vi "WPI_DashboardUpdateNames.vi"(11 "Controls on Tab":refnum<vi>[](array[refnum])) -> ()   [LabVIEW 2025]
doc: "Compare and update the captions, displayed names, of the controls on the Basic Tab. The names can be modified directly by editing on the panel, or they can be set in robot code such as is shown in Begin.vi."
uses:
  <vilib>/Rock Robotics/Network Tables/NT Read String Array.vi
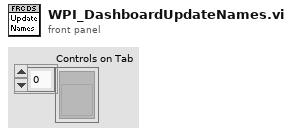
[diagram p1: front panel]
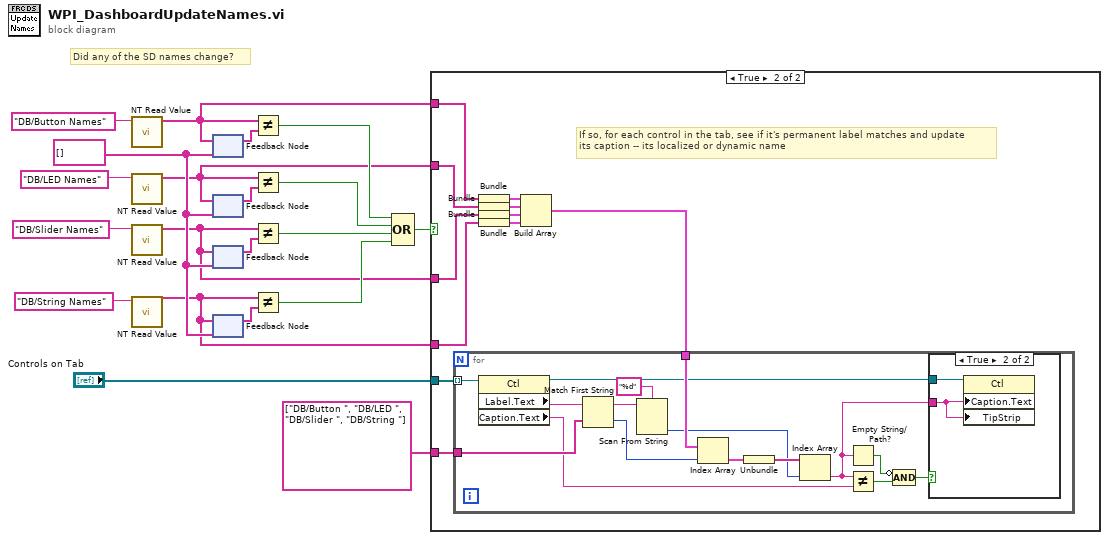
[diagram p0: block diagram]
diagram:
  w13 = string[] []
  # "Did any of the SD names change?"
  n1 = call-poly <vilib>:"NT Read Value.vi"("name"="DB/Button Names" ("Name")) -> ("value"=w7:string[])  [unwired: 8 in, 2 out]
  n2 = call-poly <vilib>:"NT Read Value.vi"("name"="DB/LED Names" ("Name")) -> ("value"=w2:string[])  [unwired: 8 in, 2 out]
  n3 = call-poly <vilib>:"NT Read Value.vi"("name"="DB/Slider Names" ("Name")) -> ("value"=w3:string[])  [unwired: 8 in, 2 out]
  n4 = call-poly <vilib>:"NT Read Value.vi"("name"="DB/String Names" ("Name")) -> ("value"=w6:string[])  [unwired: 8 in, 2 out]
  n5 = feedback #1(w13) -> (w14:string[])
  n6 = feedback-in #1(w7) -> ()
  n7 = feedback-in #2(w2) -> ()
  n8 = feedback #2(w13) -> (w20:string[])
  n9 = feedback #3(w13) -> (w19:string[])
  n10 = feedback-in #3(w3) -> ()
  n11 = feedback #4(w13) -> (w18:string[])
  n12 = feedback-in #4(w6) -> ()
  n13 = Not Equal?(x=w7, y=w14) -> (x != y?=w12:bool)
  n14 = Not Equal?(x=w2, y=w20) -> (x != y?=w11:bool)
  n15 = Not Equal?(x=w3, y=w19) -> (x != y?=w9:bool)
  n16 = Not Equal?(x=w6, y=w18) -> (x != y?=w10:bool)
  n17 = Compound Arithmetic op=OR(w12, w11, w9, w10) -> (w17:bool)
  n18 = case shown="True" w17 {
    tunnel: "Controls on Tab" -> [_ w31]
    tunnel: string[] ["DB/Button ", "DB/LED ", "DB/Slider ", "DB/String "] -> [_ w30]
    tunnel: w7 -> [_ w22]
    tunnel: w2 -> [_ w23]
    tunnel: w6 -> [_ w24]
    tunnel: w3 -> [_ w25]
    frame False {
    }
    frame True {
      # "If so, for each control in the tab, see if it's permanent label matches and update\nits caption -- its localized or dynamic name"
      n19 = Bundle("value"=w22) -> (w29:cluster{"value":string[]})  [unwired: 1 in]
      n20 = Bundle("value"=w23) -> (w28:cluster{"value":string[]})  [unwired: 1 in]
      n21 = Bundle("value"=w25) -> (w27:cluster{"value":string[]})  [unwired: 1 in]
      n22 = Bundle("value"=w24) -> (w26:cluster{"value":string[]})  [unwired: 1 in]
      n23 = Build Array(w29, w28, w27, w26) -> (w21:cluster{"value":string[]}[])
      n24 = for {
        tunnel: w31 -> [w47] mode=indexing
        tunnel: w30 -> [w45]
        tunnel: w21 -> [w42]
        n25 = property class="Ctl"(reference=w47) -> (reference out=w33:refnum<vi>, "Label.Text"=w46:string, "Caption.Text"=w37:string)  [unwired: 1 in, 1 out]
        n26 = Match First String(2:w45, 3:w46) -> (0:w41:i32, 1:w44:string)
        n27 = Scan From String(format string="%d", input string=w44) -> (output 1=w38:i32)  [unwired: 3 in, 3 out]
        n28 = Index Array(array=w42, index=w41) -> (element=w40:cluster{"value":string[]})
        n29 = Unbundle(w40) -> ("value"=w39:string[])
        n30 = Index Array(array=w39, index=w38) -> (element=w32:string)
        n31 = Empty String/Path?(string/path=w32) -> (empty?=w36:bool)
        n32 = Not Equal?(x=w32, y=w37) -> (x != y?=w35:bool)
        n33 = Compound Arithmetic op=AND(invert w36, w35) -> (w34:bool)
        n34 = case shown="True" w34 {
          tunnel: w33 -> [_ w49]
          tunnel: w32 -> [_ w48]
          frame False {
          }
          frame True {
            n35 = property class="Ctl"(reference=w49, "Caption.Text"=w48, "TipStrip"=w48) -> ()  [unwired: 1 in, 2 out]
          }
        }
      }
    }
  }
